vi "evaluateParseXML.vi"(8 "error in":errorcluster, 9 "Default VData":variant, 10 "XML string":string, 11 "reference in":refnum<class "EasyXML_XML_Subset_Source_Tests.lvclass">) -> (0 "error out":errorcluster, 1 "LabVIEW Data":variant, 3 "reference out":refnum<class "EasyXML_XML_Subset_Source_Tests.lvclass">)   [LabVIEW 2013, in "EasyXML_XML_Subset_Source_Tests.lvclass"]
uses:
  EasyXML_XML_Subset_Source_Tests.lvclass
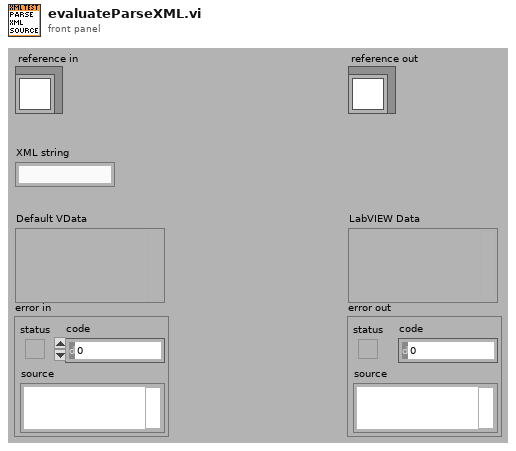
[diagram p1: front panel]
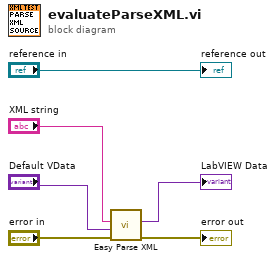
[diagram p0: block diagram]
diagram:
  n1 = call "Easy Parse XML.vi"("error in (no error)"="error in", "LabVIEW Data (Type)"="Default VData", "XML String"="XML string") -> ("error out"=→"error out":errorcluster, "LabVIEW Data"=→"LabVIEW Data":variant)  [unwired: 7 in]
  "reference out" <- "reference in"
